vi "Write Reservation Group.vi"(8 "error in (no error)":errorcluster, 10 "Reservation Group":string, 11 "SLSC Switch Init Parameters in":refnum<class "NI-SWITCH Init Parameters.lvclass">=refnum) -> (0 "error out":errorcluster, 3 "SLSC Switch Init Parameters out":refnum<class "NI-SWITCH Init Parameters.lvclass">)   [LabVIEW 2017, in "NI-SWITCH Messaging.lvlib" / "NI-SWITCH Init Parameters.lvclass"]
uses:
  NI-SWITCH Init Parameters.lvclass
  NI-SWITCH Init Parameters.lvclass/NI-SWITCH Init Parameters.ctl
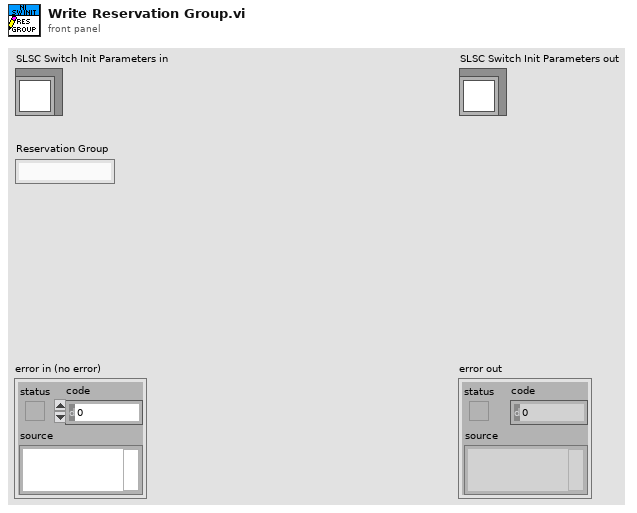
[diagram p1: front panel]
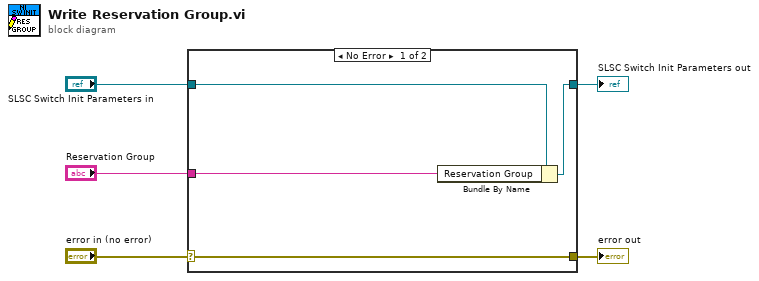
[diagram p0: block diagram]
diagram:
  n1 = case shown="No Error" "error in (no error)" {
    selector: "error in (no error)" -> [w9 w10]
    tunnel: [w9 w10] -> w4
    tunnel: [w7 w11] -> w2
    tunnel: "SLSC Switch Init Parameters in" -> [w8 w11]
    tunnel: "Reservation Group" -> [w6 _]
    frame No Error {
      n2 = Bundle By Name(cluster=w8, "Reservation Group"=w6) -> (w7:refnum<class "NI-SWITCH Init Parameters.lvclass">)
    }
    frame Error {
    }
  }
  "error out" <- w4
  "SLSC Switch Init Parameters out" <- w2
